vi "Teleop.vi"(10 "Match Info":T1={"Autonomous Elapsed Seconds"=0.0, "TeleOp Elapsed Seconds"=0.0, "Disabled Elapsed Seconds"=0.0, "Visited Autonomous"=FALSE, "Visited TeleOp"=FALSE, "Visited Disabled"=FALSE, "Autonomous Settings"={"Autonomous Style"=enum."Independent", "VI Refnum"=refnum}}, 11 "Call Context":T2) -> ()   [LabVIEW 2014]
doc: "This VI is called for each TeleOp packet received from the DS where the robot is not disabled. It is often used to read from the joysticks and update I/O or to update setpoints for timed control loops. It should complete and return within 20 milliseconds or it may miss DS packets."
uses:
  <vilib>/Rock Robotics/WPI/DriverStation/WPI_DriverStationDerivedRobotMode.ctl
  <vilib>/Rock Robotics/WPI/DriverStation/WPI_DriverStationMatch Info.ctl
  <vilib>/Rock Robotics/WPI/Joystick/WPI_JoystickGetSetRefNum.vi
  Robot Global Data.vi
  <vilib>/Rock Robotics/WPI/RobotDrive/WPI_RobotDriveGetSetRefNum.vi
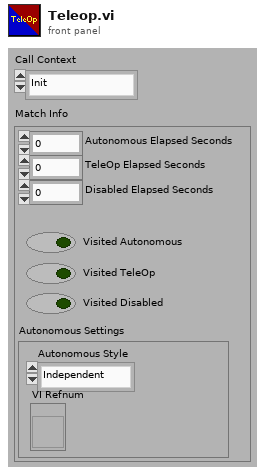
[diagram p1: front panel]
types:
  T1 = typedef "WPI_DriverStationMatch Info.ctl" = cluster{"Autonomous Elapsed Seconds":dbl, "TeleOp Elapsed Seconds":dbl, "Disabled Elapsed Seconds":dbl, "Visited Autonomous":bool, "Visited TeleOp":bool, "Visited Disabled":bool, "Autonomous Settings":cluster{"Autonomous Style":enum16{"Iterative", "Independent"}, "VI Refnum":refnum<vi>}}
  T2 = typedef "WPI_DriverStationDerivedRobotMode.ctl" = enum16{"Init", "Execute", "Stop"}
  T3 = enum16{"Tank Exp low cbd", "Tank Normal", "Limite de aceleração", "Tank exp low sqrd", "Remover deadband", "Corrige tensão"}
  T4 = typedef "WPI_JoystickDevRef.ctl" = cluster{"Device":T5}
  T5 = typedef "WPI_JoystickDeviceEnum.ctl" = enum16{"USB 0", "USB 1", "USB 2", "USB 3", "USB 4", "USB 5"}
  T6 = cluster{"Axes[0]":dbl, "Axes[1]":dbl, "Axes[2]":dbl, "Axes[3]":dbl, "Axes[4]":dbl, "Axes[5]":dbl, "Axes[6]":dbl, "Axes[7]":dbl, "Axes[8]":dbl}
  T7 = typedef "WPI_RobotDriveDevRef.ctl" = cluster{"DevStatus":errorcluster, "Motors[]":T8[], "Square Inputs":bool, "Max Output":dbl}
  T8 = typedef "WPI_MotorControlDeviceRef.ctl" = cluster{"DeviceStatus":errorcluster, "Type":T9, "PWM":cluster{"Controller":T10, "PWM Channel":T11, "DeadBand":T12}, "CAN":cluster{"Device Number":u8, "Control Mode":T13, "Semaphore":T14, "Max Vout":dbl, "TalonSRX Control Mode":T15}, "Invert":bool, "TransformRef":T16, "InvTransformRef":T16}
  T9 = typedef "WPI_MotorControlType.ctl" = enum16{"PWM", "CAN", "CANTalonSRX"}
  T10 = typedef "FPGA_TypedefDigitalModule.ctl" = enum16{"Controller 1"}
  T11 = typedef "FPGA_DIOPWMChannel.ctl" = enum8{"PWM 0", "PWM 1", "PWM 2", "PWM 3", "PWM 4", "PWM 5", "PWM 6", "PWM 7", "PWM 8", "PWM 9", "PWM MXP 0", "PWM MXP 1", "PWM MXP 2", "PWM MXP 3", "PWM MXP 4", "PWM MXP 5", "PWM MXP 6", "PWM MXP 7", "PWM MXP 8", "PWM MXP 9", "Invalid"}
  T12 = typedef "WPI_PWMDeadband.ctl" = cluster{"Name":string, "maxPositivePwm":i32, "minPositivePwm":i32, "centerPwm":i32, "maxNegativePwm":i32, "minNegativePwm":i32, "angularRange":u16}
  T13 = typedef "WPI_CANJaguar_ControlMode.ctl" = enum8{"Percent VBus", "Current", "Speed", "Position", "Voltage"}
  T14 = typedef "Semaphore RefNum" = refnum<k1>
  T15 = typedef "WPI_CANTalonSRX_APIControlMode.ctl" = enum8{"Percent VBus", "Speed", "Position", "Slave", "Unchanged / Invalid"}
  T16 = typedef "WPI_PWMTransform_ConPane.ctl" = refnum<vi>
  T17 = cluster{"POVs[0]":i16, "POVs[1]":i16, "POVs[2]":i16, "POVs[3]":i16, "POVs[4]":i16, "POVs[5]":i16, "POVs[6]":i16, "POVs[7]":i16, "POVs[8]":i16}
  T18 = cluster{"Buttons[0]":bool, "Buttons[1]":bool, "Buttons[2]":bool, "Buttons[3]":bool, "Buttons[4]":bool, "Buttons[5]":bool, "Buttons[6]":bool, "Buttons[7]":bool, "Buttons[8]":bool}
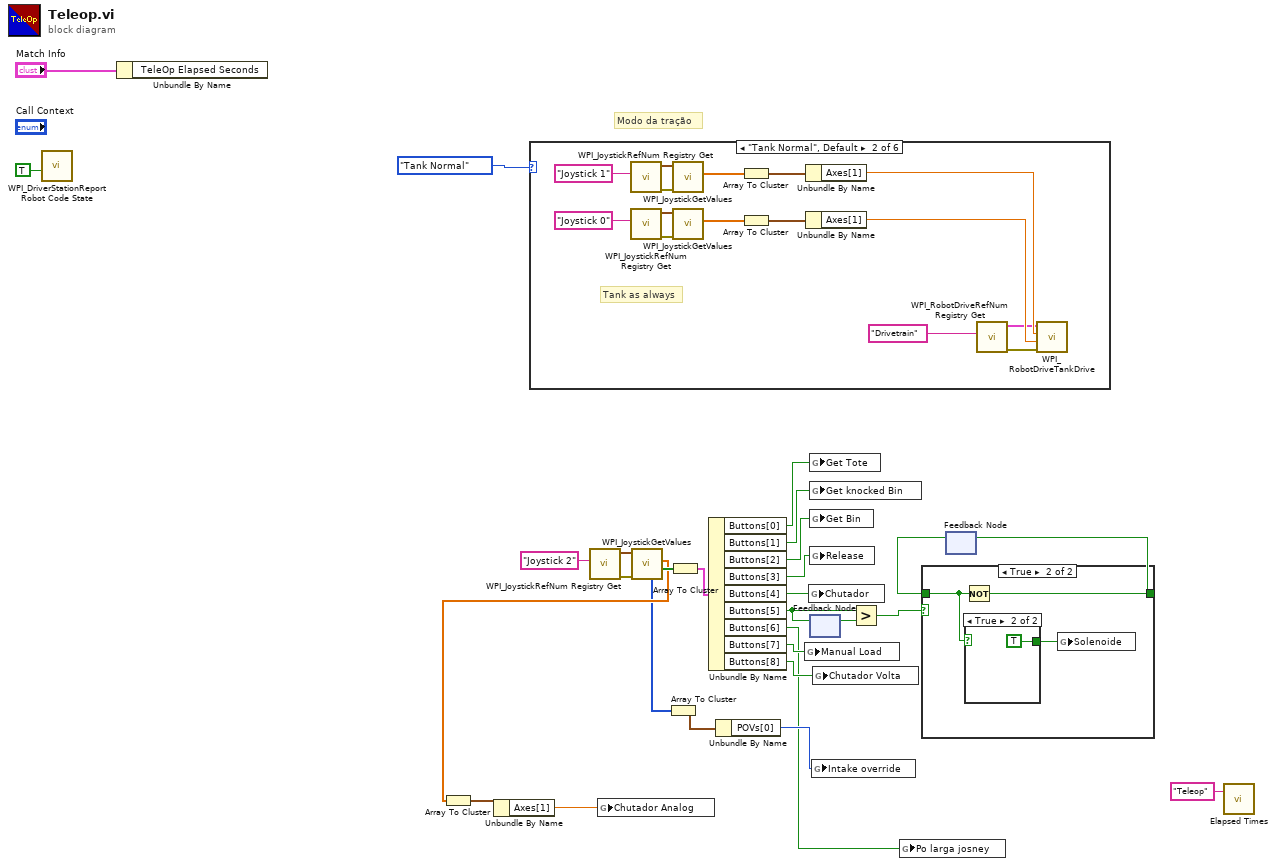
[diagram p0: block diagram]
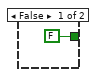
[diagram p3: hidden frame]
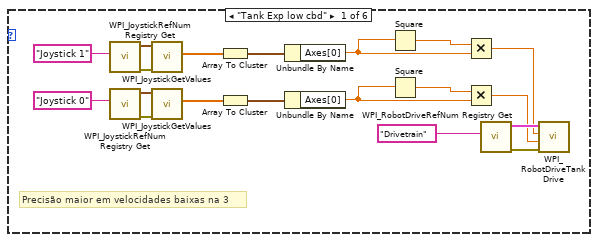
[diagram p4: hidden frame]
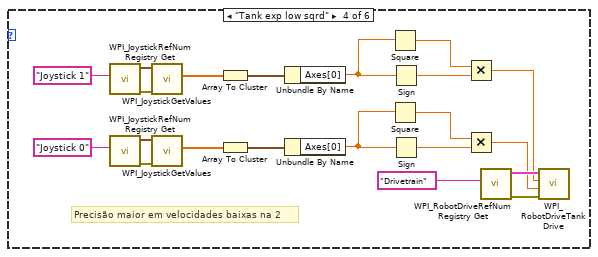
[diagram p6: hidden frame]
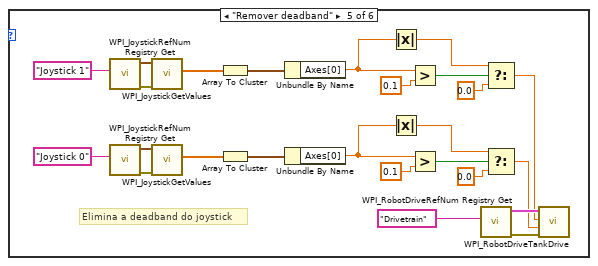
[diagram p7: hidden frame]
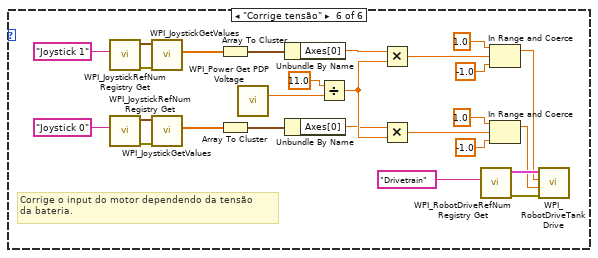
[diagram p8: hidden frame]
diagram:
  # "Modo da tração"
  n1 = call <vilib>:"WPI_DriverStationReport Robot Code State.vi"("TeleOp"=TRUE ("Autonomous")) -> ()  [unwired: 10 in, 1 out]
  n2 = Unbundle By Name("Match Info") -> ()  [unwired: 1 out]
  n3 = case shown="\"Tank Normal\", Default" T3."Tank Normal" {
    frame "Tank Exp low cbd" {
      # "Precisão maior em velocidades baixas na 3"
      n4 = call <vilib>:"WPI_JoystickRefNum Registry Get.vi"("refnum name"="Joystick 1") -> ("error out"=w46:errorcluster, "JoystickDevRef"=w47:T4)  [unwired: 9 in]
      n5 = call <vilib>:"WPI_JoystickRefNum Registry Get.vi"("refnum name"="Joystick 0") -> ("error out"=w39:errorcluster, "JoystickDevRef"=w38:T4)  [unwired: 9 in]
      n6 = call <vilib>:"WPI_JoystickGetValues.vi"("error in (no error)"=w46, "JoystickDevRef"=w47) -> ("Axes"=w44:dbl[])  [unwired: 5 in, 4 out]
      n7 = call <vilib>:"WPI_JoystickGetValues.vi"("error in (no error)"=w39, "JoystickDevRef"=w38) -> ("Axes"=w41:dbl[])  [unwired: 5 in, 4 out]
      n8 = Array To Cluster(array=w44) -> (cluster=w43:T6)
      n9 = Array To Cluster(array=w41) -> (cluster=w42:T6)
      n10 = Unbundle By Name(w43) -> ("Axes[0]"=w33:dbl)
      n11 = Unbundle By Name(w42) -> ("Axes[0]"=w30:dbl)
      n12 = Square(x=w33) -> (x^2=w34:dbl)
      n13 = Square(x=w30) -> (x^2=w31:dbl)
      n14 = Multiply(x=w34, y=w33) -> (x*y=w32:dbl)
      n15 = Multiply(x=w31, y=w30) -> (x*y=w29:dbl)
      n16 = call <vilib>:"WPI_RobotDriveRefNum Registry Get.vi"("refnum name"="Drivetrain") -> ("error out"=w36:errorcluster, "RobotDriveDevRef"=w35:T7)  [unwired: 9 in]
      n17 = call <vilib>:"WPI_RobotDriveTankDrive.vi"("error in (no error)"=w36, "Right axis value"=w29, "Left axis value"=w32, "RobotDriveDevRef"=w35) -> ()  [unwired: 5 in, 3 out]
    }
    frame "Tank Normal", Default {
      # "Tank as always"
      n18 = call <vilib>:"WPI_JoystickRefNum Registry Get.vi"("refnum name"="Joystick 1") -> ("error out"=w59:errorcluster, "JoystickDevRef"=w60:T4)  [unwired: 9 in]
      n19 = call <vilib>:"WPI_JoystickRefNum Registry Get.vi"("refnum name"="Joystick 0") -> ("error out"=w52:errorcluster, "JoystickDevRef"=w51:T4)  [unwired: 9 in]
      n20 = call <vilib>:"WPI_JoystickGetValues.vi"("error in (no error)"=w59, "JoystickDevRef"=w60) -> ("Axes"=w57:dbl[])  [unwired: 5 in, 4 out]
      n21 = call <vilib>:"WPI_JoystickGetValues.vi"("error in (no error)"=w52, "JoystickDevRef"=w51) -> ("Axes"=w54:dbl[])  [unwired: 5 in, 4 out]
      n22 = Array To Cluster(array=w57) -> (cluster=w56:T6)
      n23 = Array To Cluster(array=w54) -> (cluster=w55:T6)
      n24 = Unbundle By Name(w56) -> ("Axes[1]"=w62:dbl)
      n25 = Unbundle By Name(w55) -> ("Axes[1]"=w61:dbl)
      n26 = call <vilib>:"WPI_RobotDriveRefNum Registry Get.vi"("refnum name"="Drivetrain") -> ("error out"=w49:errorcluster, "RobotDriveDevRef"=w48:T7)  [unwired: 9 in]
      n27 = call <vilib>:"WPI_RobotDriveTankDrive.vi"("error in (no error)"=w49, "Right axis value"=w61, "Left axis value"=w62, "RobotDriveDevRef"=w48) -> ()  [unwired: 5 in, 3 out]
    }
    frame "Limite de aceleração" {
    }
    frame "Tank exp low sqrd" {
      # "Precisão maior em velocidades baixas na 2"
      n28 = call <vilib>:"WPI_JoystickRefNum Registry Get.vi"("refnum name"="Joystick 1") -> ("error out"=w82:errorcluster, "JoystickDevRef"=w83:T4)  [unwired: 9 in]
      n29 = call <vilib>:"WPI_JoystickRefNum Registry Get.vi"("refnum name"="Joystick 0") -> ("error out"=w75:errorcluster, "JoystickDevRef"=w74:T4)  [unwired: 9 in]
      n30 = call <vilib>:"WPI_JoystickGetValues.vi"("error in (no error)"=w82, "JoystickDevRef"=w83) -> ("Axes"=w80:dbl[])  [unwired: 5 in, 4 out]
      n31 = call <vilib>:"WPI_JoystickGetValues.vi"("error in (no error)"=w75, "JoystickDevRef"=w74) -> ("Axes"=w77:dbl[])  [unwired: 5 in, 4 out]
      n32 = Array To Cluster(array=w80) -> (cluster=w79:T6)
      n33 = Array To Cluster(array=w77) -> (cluster=w78:T6)
      n34 = Unbundle By Name(w79) -> ("Axes[0]"=w70:dbl)
      n35 = Unbundle By Name(w78) -> ("Axes[0]"=w65:dbl)
      n36 = Square(x=w70) -> (x^2=w68:dbl)
      n37 = Square(x=w65) -> (x^2=w64:dbl)
      n38 = Sign(1:w70) -> (0:w69:dbl)
      n39 = Sign(1:w65) -> (0:w66:dbl)
      n40 = Multiply(x=w68, y=w69) -> (x*y=w67:dbl)
      n41 = Multiply(x=w64, y=w66) -> (x*y=w63:dbl)
      n42 = call <vilib>:"WPI_RobotDriveRefNum Registry Get.vi"("refnum name"="Drivetrain") -> ("error out"=w72:errorcluster, "RobotDriveDevRef"=w71:T7)  [unwired: 9 in]
      n43 = call <vilib>:"WPI_RobotDriveTankDrive.vi"("error in (no error)"=w72, "Right axis value"=w63, "Left axis value"=w67, "RobotDriveDevRef"=w71) -> ()  [unwired: 5 in, 3 out]
    }
    frame "Remover deadband" {
      # "Elimina a deadband do joystick"
      n44 = call <vilib>:"WPI_JoystickRefNum Registry Get.vi"("refnum name"="Joystick 1") -> ("error out"=w107:errorcluster, "JoystickDevRef"=w108:T4)  [unwired: 9 in]
      n45 = call <vilib>:"WPI_JoystickRefNum Registry Get.vi"("refnum name"="Joystick 0") -> ("error out"=w100:errorcluster, "JoystickDevRef"=w99:T4)  [unwired: 9 in]
      n46 = call <vilib>:"WPI_JoystickGetValues.vi"("error in (no error)"=w107, "JoystickDevRef"=w108) -> ("Axes"=w105:dbl[])  [unwired: 5 in, 4 out]
      n47 = call <vilib>:"WPI_JoystickGetValues.vi"("error in (no error)"=w100, "JoystickDevRef"=w99) -> ("Axes"=w102:dbl[])  [unwired: 5 in, 4 out]
      n48 = Array To Cluster(array=w105) -> (cluster=w104:T6)
      n49 = Array To Cluster(array=w102) -> (cluster=w103:T6)
      n50 = Unbundle By Name(w104) -> ("Axes[0]"=w91:dbl)
      n51 = Unbundle By Name(w103) -> ("Axes[0]"=w86:dbl)
      n52 = Absolute Value(x=w91) -> (abs(x)=w94:dbl)
      n53 = Absolute Value(x=w86) -> (abs(x)=w87:dbl)
      n54 = Greater?(x=w91, y=0.1) -> (0:w95:bool)
      n55 = Greater?(x=w86, y=0.1) -> (0:w88:bool)
      n56 = call <vilib>:"WPI_RobotDriveRefNum Registry Get.vi"("refnum name"="Drivetrain") -> ("error out"=w97:errorcluster, "RobotDriveDevRef"=w96:T7)  [unwired: 9 in]
      n57 = Select(t=w94, s=w95, f=0.0) -> (s? t:f=w90:dbl)
      n58 = Select(t=w87, s=w88, f=0.0) -> (s? t:f=w84:dbl)
      n59 = call <vilib>:"WPI_RobotDriveTankDrive.vi"("error in (no error)"=w97, "Right axis value"=w84, "Left axis value"=w90, "RobotDriveDevRef"=w96) -> ()  [unwired: 5 in, 3 out]
    }
    frame "Corrige tensão" {
      # "Corrige o input do motor dependendo da tensão\nda bateria."
      n60 = call <vilib>:"WPI_JoystickRefNum Registry Get.vi"("refnum name"="Joystick 1") -> ("error out"=w133:errorcluster, "JoystickDevRef"=w134:T4)  [unwired: 9 in]
      n61 = call <vilib>:"WPI_JoystickRefNum Registry Get.vi"("refnum name"="Joystick 0") -> ("error out"=w126:errorcluster, "JoystickDevRef"=w125:T4)  [unwired: 9 in]
      n62 = call <vilib>:"WPI_JoystickGetValues.vi"("error in (no error)"=w133, "JoystickDevRef"=w134) -> ("Axes"=w131:dbl[])  [unwired: 5 in, 4 out]
      n63 = call <vilib>:"WPI_JoystickGetValues.vi"("error in (no error)"=w126, "JoystickDevRef"=w125) -> ("Axes"=w128:dbl[])  [unwired: 5 in, 4 out]
      n64 = Array To Cluster(array=w131) -> (cluster=w130:T6)
      n65 = Array To Cluster(array=w128) -> (cluster=w129:T6)
      n66 = call <vilib>:"WPI_Power Get PDP Voltage.vi"() -> ("voltage (V)"=w116:dbl)  [unwired: 14 in, 1 out]
      n67 = Unbundle By Name(w130) -> ("Axes[0]"=w121:dbl)
      n68 = Unbundle By Name(w129) -> ("Axes[0]"=w110:dbl)
      n69 = Divide(x=11.0, y=w116) -> (x/y=w111:dbl)
      n70 = Multiply(x=w121, y=w111) -> (x*y=w120:dbl)
      n71 = Multiply(x=w110, y=w111) -> (x*y=w112:dbl)
      n72 = call <vilib>:"WPI_RobotDriveRefNum Registry Get.vi"("refnum name"="Drivetrain") -> ("error out"=w123:errorcluster, "RobotDriveDevRef"=w122:T7)  [unwired: 9 in]
      n73 = In Range and Coerce(upper limit=1.0, x=w120, lower limit=-1.0) -> (coerced(x)=w117:dbl)  [unwired: 1 out]
      n74 = In Range and Coerce(upper limit=1.0, x=w112, lower limit=-1.0) -> (coerced(x)=w109:dbl)  [unwired: 1 out]
      n75 = call <vilib>:"WPI_RobotDriveTankDrive.vi"("error in (no error)"=w123, "Right axis value"=w109, "Left axis value"=w117, "RobotDriveDevRef"=w122) -> ()  [unwired: 5 in, 3 out]
    }
  }
  n76 = call <vilib>:"WPI_JoystickRefNum Registry Get.vi"("refnum name"="Joystick 2") -> ("error out"=w24:errorcluster, "JoystickDevRef"=w25:T4)  [unwired: 9 in]
  n77 = call <vilib>:"WPI_JoystickGetValues.vi"("error in (no error)"=w24, "JoystickDevRef"=w25) -> ("Buttons"=w21:bool[], "Axes"=w8:dbl[], "POVs"=w4:i16[])  [unwired: 5 in, 2 out]
  n78 = Array To Cluster(array=w8) -> (cluster=w9:T6)
  n79 = Unbundle By Name(w9) -> ("Axes[1]"=w6:dbl)
  n80 = global write "Robot Global Data.vi" "Chutador Analog"(w6) -> ()
  n81 = Array To Cluster(array=w4) -> (cluster=w3:T17)
  n82 = Array To Cluster(array=w21) -> (cluster=w22:T18)
  n83 = Unbundle By Name(w22) -> ("Buttons[0]"=w16:bool, "Buttons[1]"=w20:bool, "Buttons[2]"=w19:bool, "Buttons[3]"=w18:bool, "Buttons[4]"=w17:bool, "Buttons[5]"=w15:bool, "Buttons[6]"=w1:bool, "Buttons[7]"=w10:bool, "Buttons[8]"=w7:bool)
  n84 = Unbundle By Name(w3) -> ("POVs[0]"=w2:i16)
  n85 = global write "Robot Global Data.vi" "Manual Load"(w10) -> ()
  n86 = global write "Robot Global Data.vi" "Chutador"(w17) -> ()
  n87 = global write "Robot Global Data.vi" "Get Tote"(w16) -> ()
  n88 = global write "Robot Global Data.vi" "Get knocked Bin"(w20) -> ()
  n89 = global write "Robot Global Data.vi" "Get Bin"(w19) -> ()
  n90 = global write "Robot Global Data.vi" "Release"(w18) -> ()
  n91 = feedback-in #1(w15) -> ()
  n92 = feedback #1() -> (w14:bool)  [unwired: 1 in]
  n93 = global write "Robot Global Data.vi" "Intake override"(w2) -> ()
  n94 = global write "Robot Global Data.vi" "Chutador Volta"(w7) -> ()
  n95 = Greater?(x=w15, y=w14) -> (0:w13:bool)
  n96 = global write "Robot Global Data.vi" "Po larga josney"(w1) -> ()
  n97 = feedback #2() -> (w12:bool)  [unwired: 1 in]
  n98 = case shown="True" w13 {
    tunnel: [w135 w138] -> w11
    tunnel: w12 -> [w135 w137]
    frame False {
    }
    frame True {
      n99 = Not(x=w137) -> (.not. x?=w138:bool)
      n100 = case shown="True" w137 {
        tunnel: [FALSE TRUE] -> w136
        frame False {
        }
        frame True {
        }
      }
      n101 = global write "Robot Global Data.vi" "Solenoide"(w136) -> ()
    }
  }
  n102 = feedback-in #2(w11) -> ()
  n103 = call "Elapsed Times.vi"("Call Name"="Teleop") -> ()  [unwired: 2 in, 1 out]
